vi "AMZ_S3_APIHLP_Parse Initiate Multipart Upload Result.vi"(8 "error in (no error)":errorcluster, 10 "Response body":string) -> (0 "error out":errorcluster, 3 "InitiateMultipartUploadResult":T1)   [LabVIEW 2015, in "LV Interface for Amazon S3.lvlib"]
uses:
  LV Interface for Amazon S3.lvlib
  Typedefs/AMZ_S3_API_InitiateMultipartUploadResult.ctl
  XML Parser/XML Parser.lvlib
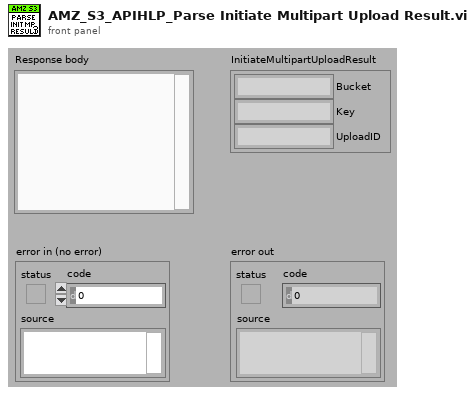
[diagram p1: front panel]
types:
  T1 = typedef "LV Interface for Amazon S3.lvlib/AMZ_S3_API_InitiateMultipartUploadResult.ctl" = cluster{"Bucket":string, "Key":string, "UploadID":string}
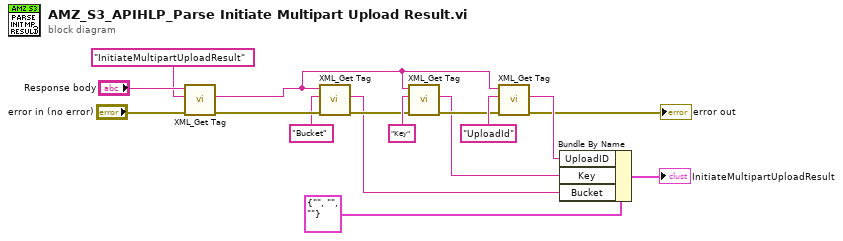
[diagram p0: block diagram]
diagram:
  n1 = call "XML_Get Tag.vi"("error in (no error)"="error in (no error)", "Tag name"="InitiateMultipartUploadResult", "XML String in"="Response body") -> ("error out"=w13:errorcluster, "Tag value"=w7:string)  [unwired: 4 in, 3 out]
  n2 = call "XML_Get Tag.vi"("error in (no error)"=w13, "Tag name"="Bucket", "XML String in"=w7) -> ("error out"=w10:errorcluster, "Tag value"=w5:string)  [unwired: 4 in, 3 out]
  n3 = call "XML_Get Tag.vi"("error in (no error)"=w10, "Tag name"="Key", "XML String in"=w7) -> ("error out"=w8:errorcluster, "Tag value"=w4:string)  [unwired: 4 in, 3 out]
  n4 = call "XML_Get Tag.vi"("error in (no error)"=w8, "Tag name"="UploadId", "XML String in"=w7) -> ("error out"=→"error out":errorcluster, "Tag value"=w3:string)  [unwired: 4 in, 3 out]
  n5 = Bundle By Name(cluster=T1 {"Bucket"="", "Key"="", "UploadID"=""} ("InitiateMultipartUploadResult"), "UploadID"=w3, "Key"=w4, "Bucket"=w5) -> (→"InitiateMultipartUploadResult":T1)
